vi "Write Icon (BitMap).vi"(8 "error in (no error)":errorcluster, 9 "Icon (BitMap) True":refnum<class "BitMap.lvclass">, 10 "Icon (BitMap) False":refnum<class "BitMap.lvclass">, 11 "Control in":refnum<class "Control.lvclass">) -> (0 "error out":errorcluster, 3 "Control out":refnum<class "Control.lvclass">)   [LabVIEW 2012, in "Control.lvclass"]
uses:
  Control.lvclass
  <userlib>/BitMan/BitMap class/BitMap.lvclass
  Control.lvclass/Control.ctl
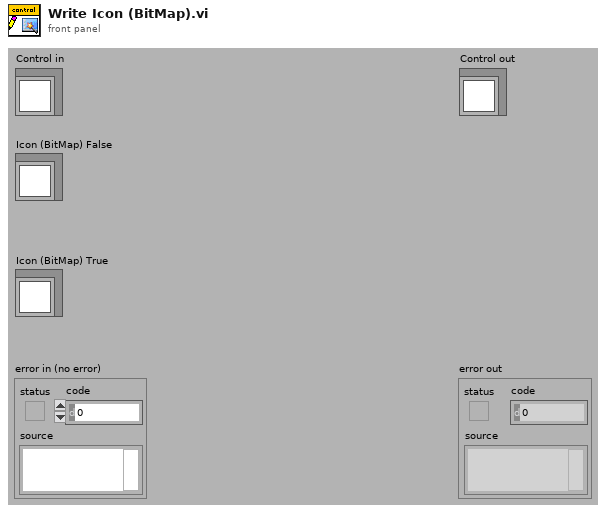
[diagram p1: front panel]
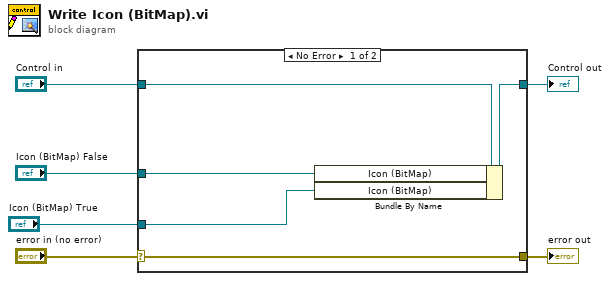
[diagram p0: block diagram]
diagram:
  n1 = case shown="No Error" "error in (no error)" {
    selector: "error in (no error)" -> [w11 w12]
    tunnel: [w11 w12] -> w5
    tunnel: [w9 w13] -> w3
    tunnel: "Control in" -> [w10 w13]
    tunnel: "Icon (BitMap) False" -> [w8 _]
    tunnel: "Icon (BitMap) True" -> [w7 _]
    frame No Error {
      n2 = Bundle By Name(cluster=w10, "Icon (BitMap)"=w8, "Icon (BitMap)"=w7) -> (w9:refnum<class "Control.lvclass">)
    }
    frame Error {
    }
  }
  "error out" <- w5
  "Control out" <- w3
